vi "Send Log API.vi"(8 "error in (no error)":errorcluster, 11 "Data":T1 {"Time Stamp" format="%<%x %.3X>T"}) -> (0 "error out":errorcluster)   [LabVIEW 2021, in "Error_Manager.lvlib" / "LogRotate.lvclass"]
uses:
  LogRotate.lvclass
  LogData.ctl
  LogRotate.lvclass/LogRotate.ctl
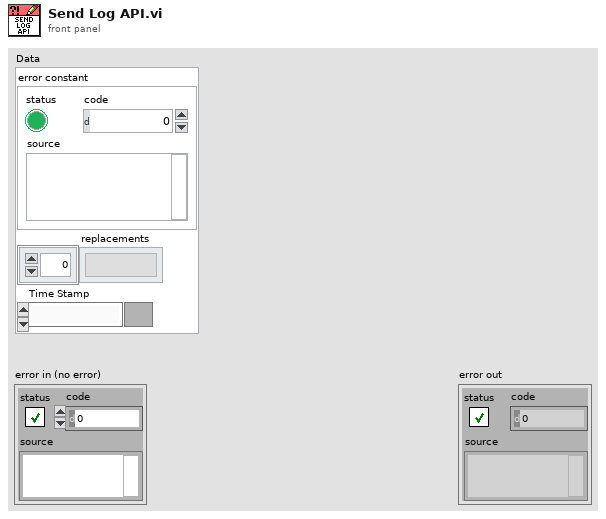
[diagram p1: front panel]
types:
  T1 = typedef "Error_Manager.lvlib/LogRotate.lvclass/LogData.ctl" = cluster{"error constant":errorcluster, "replacements":string[], "Time Stamp":timestamp}
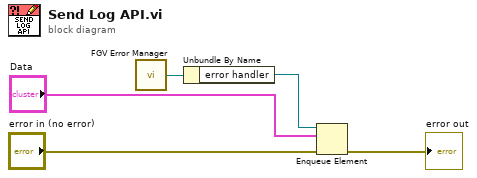
[diagram p0: block diagram]
diagram:
  n1 = call "FGV Error Manager.vi"() -> ("error_manager out"=w4:refnum<class "LogRotate.lvclass">)  [unwired: 1 in]
  n2 = Unbundle By Name(w4) -> ("error handler"=w2:refnum<queue>)
  n3 = Enqueue Element(queue=w2, element="Data", error in (no error)="error in (no error)") -> (error out=→"error out":errorcluster)  [unwired: 1 in, 2 out]
